vi "BenchC2_DEV_v15_3.vi"() -> ()   [LabVIEW 2017]
uses:
  x64/Debug/BERTTA.dll
panel:
  out "Started:":string
  in  "SHUTDOWN":bool
  in  "MASTER CONTROL":bool
  in  "Tab Control":T1(tab)
  out "Output File":path caption="selected path"
  in  "Browse folder":path=path "" caption="start path"
  in  "Read Seq":bool
  in  "Save Seq":bool
  in  "Configuration file":path caption="Filename"
  in  "OK Button 2":bool
  out "Boolean":bool
  in  "User (initials)":string
  in  "Project name":string
  in  "Description":string
  out "Led11 12":bool
  out "Led11 11":bool
  out "PUMP1":bool
  out "Target amount":dbl format="Target amount:        %#_g"
  out "Scale weight":dbl format="Scale weight:     %#_4g"
  out "Amount now":dbl format="Amount now:      %#_4g"
  out "Flow rate":dbl format="Flow rate:                   %#_4g"
  out "Time to target":dbl format="Time to target:     %<%H:%M:%S>t"
  out "Current step":dbl format="Current step:              %#_g"
  out "Target":dbl format="Target:                %#_4g"
  out "Amount now":dbl format="Amount now:    %#_4g"
  out "Amount now":dbl
  out "Target":dbl
  out "Current step":dbl
  out "Time to target":dbl format="%<%H:%M:%S>t"
  out "Flow rate":dbl
  out "Amount now":dbl
  out "Scale weight":dbl
  out "Target amount":dbl
  out "PUMP2":bool
  out "Sensor OK 6":bool
  out "Sensor OK 5":bool
  out "Sensor OK 4":bool
  out "Sensor OK 3":bool
  in  "OK Button":bool
  in  "Add comment":string
  out "Tr":dbl format="Tr:              %#_4g"
  out "Tj in":dbl format="Tj in:        %#_4g"
  out "Tj out":dbl format="Tj out:        %#_4g"
  out "T set":dbl format="T set:          %#_g"
  out "Current step":i32 format="Current step:  %.0f"
  out "RPM":dbl format="RPM:          %#_g"
  out "Torque 2":dbl format="Torque:      %#_g"
  out "PUMP3":bool
  out "Target amount":dbl
  out "Scale weight":dbl
  out "Amount now":dbl
  out "Flow rate":dbl
  out "Time to target":dbl format="%<%H:%M:%S>t"
  out "Current step":dbl
  out "Target":dbl
  out "Amount now":dbl
  out "Waveform Chart 5":dynamicdata(graph)
  out "Waveform Chart 6":dynamicdata(graph)
  out "Waveform Chart 7":dynamicdata(graph)
  out "Led11 10":bool
  out "T external 3":dbl format="T (S2):       %#_4g"
  out "Table":string[][](table)=[["14.8.2017 18.06.59", "0,000000", "417,670000", "-0,150000", "1,000000", "22,220000", "23,366837", "23,574959", "23,985852", "23,690000", "240,000000", "4,000000", "0,000000", "397,000000", "-397,000000", "1,000000"], ["14.8.2017 18.07.06", "0,000000", "417,640000", "-0,120000", "1,000000", "22,220000", "23,763115", "23,906257", "23,985694", "23,680000", "240,000000", "4,000000", "0,000000", "397,000000", "-397,000000", "1,000000"], ["14.8.2017 18.07.13", "0,000000", "417,640000", "-0,120000", "1,000000", "22,220000", "23,965922", "24,013440", "23,984906", "23,670000", "240,000000", "4,100000", "3,000000", "397,000000", "-397,000000", "1,000000"], ["14.8.2017 18.07.21", "0,000000", "417,640000", "-0,120000", "1,000000", "22,220000", "23,943860", "23,900110", "23,987113", "23,670000", "240,000000", "4,000000", "0,000000", "397,000000", "-397,000000", "1,000000"], ["14.8.2017 18.07.28", "0,000000", "417,640000", "-0,120000", "1,000000", "22,220000", "23,736328", "23,600018", "23,989004", "23,660000", "240,000000", "4,000000", "0,000000", "397,000000", "-397,000000", "1,000000"], ["14.8.2017 18.07.36", "0,000000", "417,640000", "-0,120000", "1,000000", "22,220000", "23,480910", "23,324538", "23,991053", "23,660000", "240,000000", "4,000000", "0,000000", "397,000000", "-397,000000", "1,000000"], ["14.8.2017 18.07.43", "0,000000", "417,640000", "-0,120000", "2,000000", "22,220000", "23,195579", "23,008270", "23,999093", "23,650000", "240,000000", "4,000000", "0,000000", "397,000000", "-397,000000", "1,000000"], ["14.8.2017 18.07.51", "0,000000", "417,650000", "-417,650000", "1,000000", "22,220000", "22,862541", "22,649021", "24,003979", "23,650000", "240,000000", "4,000000", "0,000000", "397,000000", "-397,000000", "2,000000"], ["14.8.2017 18.07.58", "0,000000", "417,640000", "0,010000", "1,000000", "22,220000", "22,541353", "22,354878", "24,005398", "23,650000", "240,000000", "4,000000", "0,000000", "397,000000", "-397,000000", "1,000000"], ["14.8.2017 18.08.06", "0,000000", "417,640000", "0,010000", "1,000000", "22,220000", "22,347931", "22,253738", "24,007605", "23,640000", "240,000000", "4,100000", "0,000000", "397,000000", "-397,000000", "1,000000"], ["14.8.2017 18.08.13", "0,000000", "417,640000", "0,010000", "1,000000", "22,220000", "22,329030", "22,302102", "24,006028", "23,640000", "240,000000", "4,000000", "0,000000", "395,820000", "-395,820000", "1,000000"], ["14.8.2017 18.08.20", "0,000000", "417,640000", "0,010000", "1,000000", "22,220000", "22,466849", "22,511320", "24,002403", "23,630000", "240,000000", "4,000000", "0,000000", "395,830000", "-0,010000", "1,000000"], ["14.8.2017 18.08.28", "0,000000", "417,640000", "0,010000", "1,000000", "22,220000", "22,707062", "22,835101", "24,000984", "23,620000", "240,000000", "4,000000", "0,000000", "395,830000", "-0,010000", "1,000000"], ["14.8.2017 18.08.35", "0,000000", "417,640000", "0,010000", "1,000000", "22,220000", "23,054104", "23,232979", "24,001299", "23,600000", "240,000000", "4,000000", "0,000000", "395,830000", "-0,010000", "1,000000"], ["14.8.2017 18.08.43", "0,000000", "417,640000", "0,010000", "1,000000", "22,220000", "23,412371", "23,522793", "24,002560", "23,590000", "240,000000", "4,000000", "0,000000", "395,820000", "0,000000", "1,000000"], ["14.8.2017 18.08.51", "0,000000", "417,640000", "0,010000", "1,000000", "22,220000", "23,596247", "23,656125", "24,003821", "23,580000", "240,000000", "4,000000", "0,000000", "395,820000", "0,000000", "1,000000"]]
  out "LED_5":bool
  out "LED_4":bool
  in  "PAUSE/RUN 4":bool
  in  "TEMP RAMP":dbl[][](array[numeric])
  out "LED_3":bool
  out "LED_2":bool
  out "LED_1":bool
  out "LED_MANUAL":bool
  in  "Reset 6":bool
  in  "Manual/Ramp":bool=TRUE
  in  "Sensor selector":bool=TRUE
  in  "Tr/Tj mode selector":bool=TRUE
  out "LED STOP":bool
  in  "Failsafe":dbl=20.0 format="Failsafe temperature:            %#_g"
  out "Current temp":dbl format="Current temperature S1:       %#_4g"
  out "Sensor OK":bool
  out "T external 2":dbl format="Current temperature S2:       %#_4g"
  in  "OK Button 3":bool
  out "Waveform Chart":dynamicdata(graph)
  in  "X scale":i64(slide)=50 scale=0.0..100.0
  out "Led11 7":bool
  out "Led11 6":bool
  out "Led11 7":bool
  out "Led11 6":bool
  out "Led5 7":bool
  out "Led4 6":bool
  out "Waveform Chart 18":dynamicdata(graph)
  in  "PAUSE/RUN 3":bool
  in  "Tube select 3":u32(ring) items=["Big tube", "Double big tube", "Medium tube", "Small tube"]
  in  "Reset 8":bool
  out "Led11 9":bool
  in  "?":bool
  in  "Grams / min 3":dbl
  out "RPM 3":dbl format="%_4f"
  out "Flow rate (g/min) 3":dbl
  out "Scale reading 3":dbl
  out "Step amount now 3":dbl
  out "Total amount now 3":dbl
  out "Elapsed / step 3":dbl format="%<%H:%M:%S>t"
  out "Time to target 3":dbl format="%<%H:%M:%S>t"
  out "Led5 5":bool
  out "Led4 5":bool
  out "Led3 5":bool
  out "Led2 5":bool
  out "Led1 5":bool
  in  "PumpSeq 6":dbl[][](array[numeric])=[[0.0, 0.0, 0.0, 0.0, 0.0, 0.0, 0.0, 0.0, 0.0, 0.0], [0.0, 0.0, 0.0, 0.0, 0.0, 0.0, 0.0, 0.0, 0.0, 0.0], [0.0, 0.0, 0.0, 0.0, 0.0, 0.0, 0.0, 0.0, 0.0, 0.0], [0.0, 0.0, 0.0, 0.0, 0.0, 0.0, 0.0, 0.0, 0.0, 0.0], [0.0, 0.0, 0.0, 0.0, 0.0, 0.0, 0.0, 0.0, 0.0, 0.0], [0.0, 0.0, 0.0, 0.0, 0.0, 0.0, 0.0, 0.0, 0.0, 0.0], [0.0, 0.0, 0.0, 0.0, 0.0, 0.0, 0.0, 0.0, 0.0, 0.0], [0.0, 0.0, 0.0, 0.0, 0.0, 0.0, 0.0, 0.0, 0.0, 0.0], [0.0, 0.0, 0.0, 0.0, 0.0, 0.0, 0.0, 0.0, 0.0, 0.0], [0.0, 0.0, 0.0, 0.0, 0.0, 0.0, 0.0, 0.0, 0.0, 0.0]]
  out "Led11 8":bool
  in  "PAUSE/RUN 2":bool
  in  "Tube select 2":u32(ring) items=["Big tube", "Double big tube", "Medium tube", "Small tube"]
  out "Led11 7":bool
  in  "?":bool
  in  "Grams / min 2":dbl
  out "RPM 2":dbl format="%_4f"
  out "Flow rate (g/min) 2":dbl
  out "Scale reading 2":dbl
  out "Step amount now 2":dbl
  out "Total amount now 2":dbl
  out "Elapsed / step 2":dbl format="%<%H:%M:%S>t"
  out "Time to target 2":dbl format="%<%H:%M:%S>t"
  out "Led5 4":bool
  out "Led4 4":bool
  out "Led3 4":bool
  out "Led2 4":bool
  out "Led1 4":bool
  in  "PumpSeq 5":dbl[][](array[numeric])=[[0.0, 0.0, 0.0, 0.0, 0.0, 0.0, 0.0, 0.0, 0.0, 0.0], [0.0, 0.0, 0.0, 0.0, 0.0, 0.0, 0.0, 0.0, 0.0, 0.0], [0.0, 0.0, 0.0, 0.0, 0.0, 0.0, 0.0, 0.0, 0.0, 0.0], [0.0, 0.0, 0.0, 0.0, 0.0, 0.0, 0.0, 0.0, 0.0, 0.0], [0.0, 0.0, 0.0, 0.0, 0.0, 0.0, 0.0, 0.0, 0.0, 0.0], [0.0, 0.0, 0.0, 0.0, 0.0, 0.0, 0.0, 0.0, 0.0, 0.0], [0.0, 0.0, 0.0, 0.0, 0.0, 0.0, 0.0, 0.0, 0.0, 0.0], [0.0, 0.0, 0.0, 0.0, 0.0, 0.0, 0.0, 0.0, 0.0, 0.0], [0.0, 0.0, 0.0, 0.0, 0.0, 0.0, 0.0, 0.0, 0.0, 0.0], [0.0, 0.0, 0.0, 0.0, 0.0, 0.0, 0.0, 0.0, 0.0, 0.0]]
  out "Led11 6":bool
  in  "Reset 7":bool
  in  "PAUSE/RUN":bool
  in  "Tube select":u32(ring) items=["Big tube", "Double big tube", "Medium tube", "Small tube"]
  out "Led11 5":bool
  out "RPM":dbl format="RPM                      %_4f"
  out "Flow rate (g/min)":dbl format="Flow rate               %#_g"
  out "Scale reading":dbl format="Scale reading       %#_g"
  out "Step amount now":dbl format="Step amount       %#_g"
  out "Total amount now":dbl format="Total amount      %#_g"
  out "Elapsed / step":dbl format="Elapsed / step      %<%H:%M:%S>t"
  out "Time to target":dbl format="Time to target     %<%H:%M:%S>t"
  out "Led5 3":bool
  out "Led4 3":bool
  out "Led3 3":bool
  out "Led2 3":bool
  out "Led1 3":bool
  in  "PumpSeq 4":dbl[][](array[numeric])=[[0.0, 0.0, 0.0, 0.0, 0.0, 0.0, 0.0, 0.0, 0.0, 0.0], [0.0, 0.0, 0.0, 0.0, 0.0, 0.0, 0.0, 0.0, 0.0, 0.0], [0.0, 0.0, 0.0, 0.0, 0.0, 0.0, 0.0, 0.0, 0.0, 0.0], [0.0, 0.0, 0.0, 0.0, 0.0, 0.0, 0.0, 0.0, 0.0, 0.0], [0.0, 0.0, 0.0, 0.0, 0.0, 0.0, 0.0, 0.0, 0.0, 0.0], [0.0, 0.0, 0.0, 0.0, 0.0, 0.0, 0.0, 0.0, 0.0, 0.0], [0.0, 0.0, 0.0, 0.0, 0.0, 0.0, 0.0, 0.0, 0.0, 0.0], [0.0, 0.0, 0.0, 0.0, 0.0, 0.0, 0.0, 0.0, 0.0, 0.0], [0.0, 0.0, 0.0, 0.0, 0.0, 0.0, 0.0, 0.0, 0.0, 0.0], [0.0, 0.0, 0.0, 0.0, 0.0, 0.0, 0.0, 0.0, 0.0, 0.0]]
  in  "?":bool
  in  "Grams / min":dbl format="Manual g/min:  %#_g"
  out "Led11 4":bool
  in  "Reset 5":bool
  in  "OK Button 4":bool
  out "Waveform Chart 16":dynamicdata(graph)
  in  "OK Button 5":bool
  out "Waveform Chart 17":dynamicdata(graph)
  in  "OK Button 6":bool
  in  "PAUSE/RUN 5":bool
  in  "?":bool
  in  "Scale port":dbl=5.0
  out "Waveform Chart 15":dynamicdata(graph)
  in  "OK Button 8":bool
  in  "PAUSE/RUN 6":bool
  in  "Set RPM":i32
  in  "Remote / Manual":bool
  out "RPM":dbl
  out "Torque":dbl
  out "Waveform Chart 4":dynamicdata(graph)
  in  "OK Button 7":bool
  in  "CDAQ Temp Control":tag="cDAQ9188XT-1C3BF12Mod1"
  in  "CDAQ PAM Control":tag="cDAQ9188XT-1C3BF12Mod1"
  in  "PORT PUMP2":i32 format="PUMP 2 PORT:  %.0f"
  in  "PORT PUMP3":i32 format="PUMP 3 PORT:  %.0f"
  in  "PORT PUMP1":i32 format="PUMP 1 PORT:  %.0f"
  in  "Save PortDev":bool
  in  "LAUDA":i32 format="LAUDA PORT:  %.0f"
  in  "HEIDOLPH":i32 format="HEIDOLPH PORT:  %.0f"
  in  "SCALE1":i32 format="SCALE 1 PORT:  %.0f"
  in  "SCALE2":i32 format="SCALE 2 PORT:  %.0f"
  in  "SCALE 3":i32 format="SCALE 3 PORT:  %.0f"
  # "PUMP & SCALE 1"
  # "PUMP & SCALE 2"
  # "PUMP & SCALE 3"
  # "STEP"
  # "STEP"
  # "STEP"
  # "TOTAL"
  # "TOTAL"
  # "TOTAL"
  # "Temperature sensor:"
  # "Manual control:"
  # "MANUAL"
  # "RAMP"
  # "Temp Target       Time Target          Wait Time"
  # "STOP"
  # "g              min"
  # "g              min"
  # "g              min"
  # "PAM control"
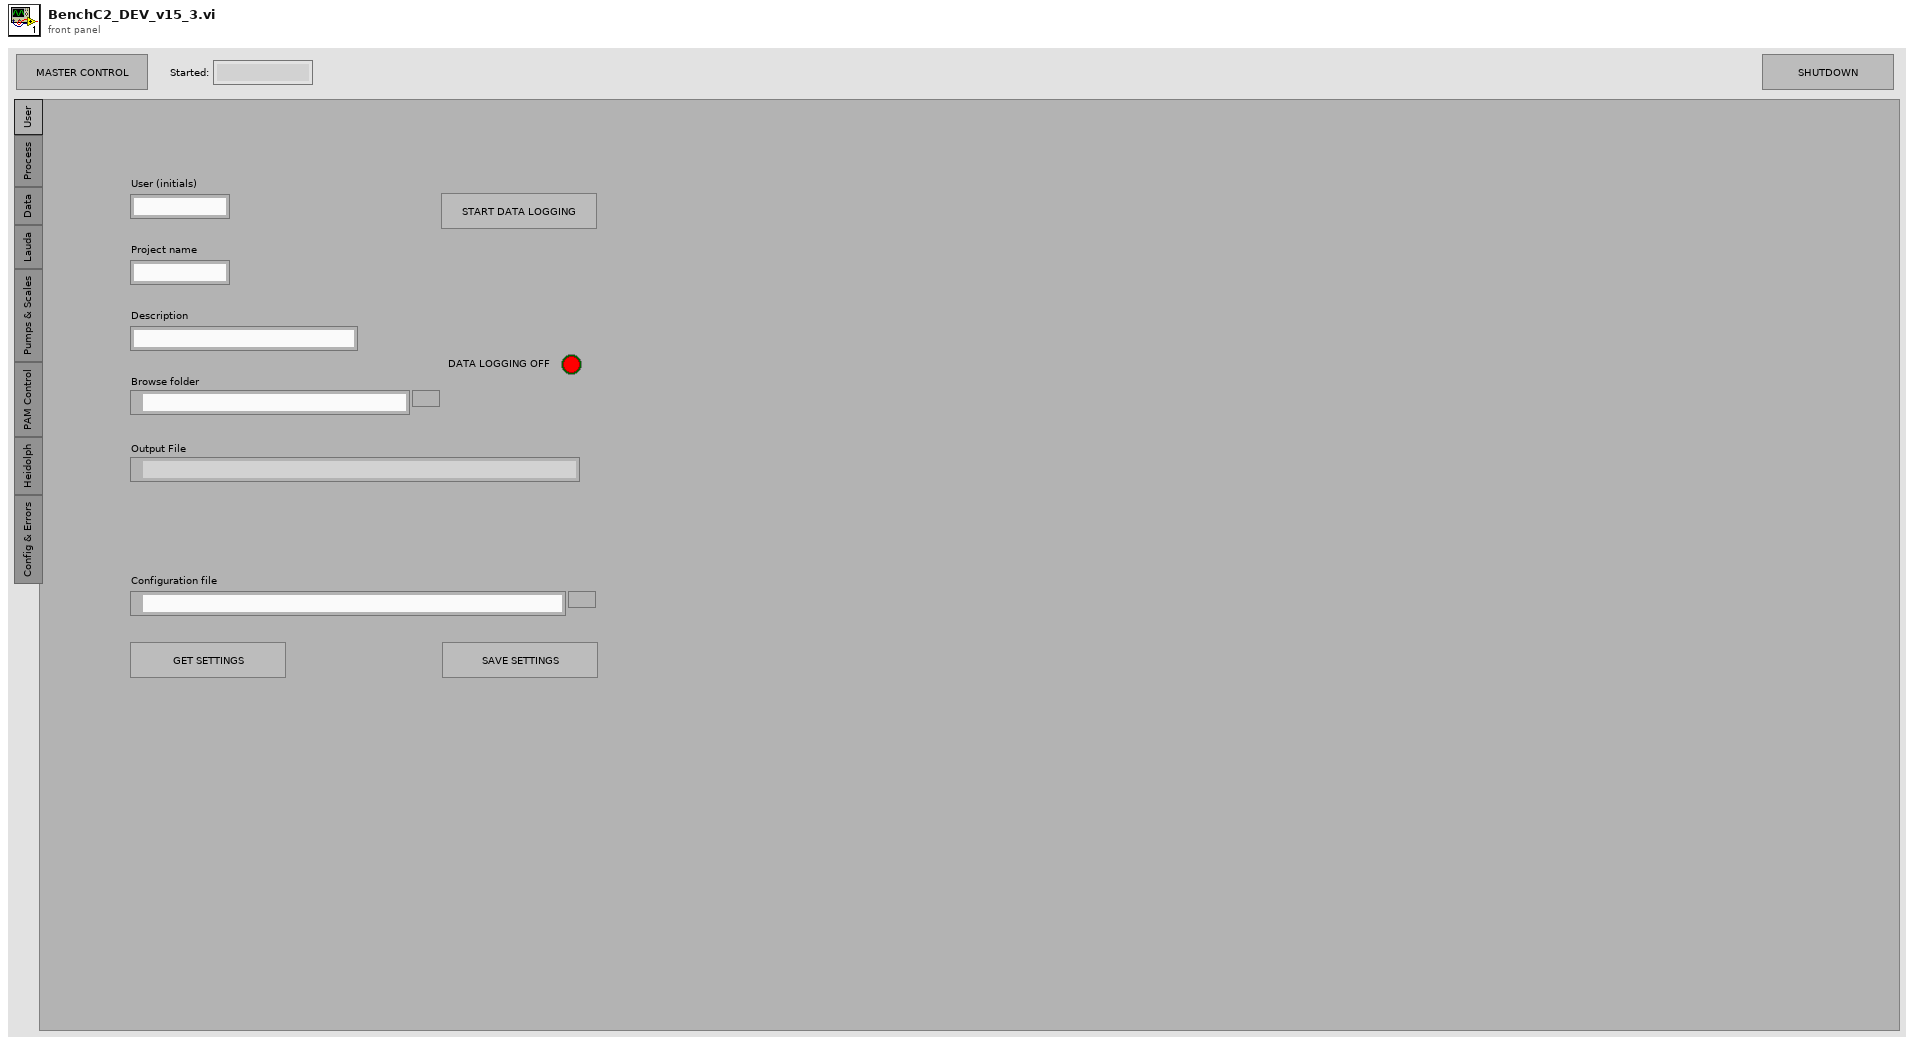
[diagram p1: front panel]
types:
  T1 = enum32{"User", "Process", "Data", "Lauda", "Pumps & Scales", "PAM Control", "Heidolph", "Config & Errors"}
diagram:
  n1 = while {
    i -> [w227]
    stop <- FALSE stop-if-true
    w31 = i64 1000 ("y")
    # "TARKISTA: negatiiviset lämpötilat, toimivatko"
    # "X-skaalaus puuttuu"
    # "SCALE & PUMP 1"
    # "SCALE & PUMP 3"
    n2 = And(x="PAUSE/RUN 6", y="MASTER CONTROL") -> (x .and. y?=w8:bool)
    n3 = feedback #1() -> (w36:dbl[][])  [unwired: 1 in]
    n4 = Select(t="TEMP RAMP", s="Reset 6", f=w36) -> (s? t:f=w37:dbl[][])
    n5 = feedback-in #1(w37) -> ()
    n6 = Initialize Array(0.0 ("element"), 5 ("dimension size"), 3 ("dimension size")) -> (w81:dbl[][])
    n7 = Select(t="Set RPM", s=w8, f=10) -> (s? t:f=w12:i32)
    n8 = Not(x="MASTER CONTROL") -> (.not. x?=w280:bool)
    n9 = Replace Array Subset(array=w81, new element=w36, index (row)=0, index (col)=0 ("disabled index (col)")) -> (w55:dbl[][])
    n10 = control-ref of="This VI"() -> (w4:refnum<vi>)
    n11 = Multiply(x="X scale", y=w31) -> (x*y=w32:i64)
    n12 = Boolean To (0,1)(Boolean=w280) -> (0, 1=w281:i16)
    n13 = Add(x=w32, y=w31) -> (x+y=w27:i64)
    n14 = for {
      N: w281 -> [_]
      n15 = Get Date/Time String(want seconds? (F)=TRUE) -> (time string=→"Started:":string)  [unwired: 2 in, 1 out]
    }
    n16 = feedback #2() -> (w30:i64)  [unwired: 1 in]
    n17 = feedback-in #2(w27) -> ()
    n18 = Boolean To (0,1)(Boolean="Sensor selector") -> (0, 1=w63:i16)
    n19 = Boolean To (0,1)(Boolean="SHUTDOWN") -> (0, 1=w2:i16)
    n20 = call "shutdown sequence.vi"("SHUTDOWN"="SHUTDOWN", "VI in"=w4) -> ()  [unwired: 10 in]
    n21 = Not Equal?(x=w30, y=w27) -> (x != y?=w29:bool)
    n22 = property on="Waveform Chart" class="WFChart (strict)"() -> ("History Data"=w34:dynamicdata[])  [unwired: 2 in, 2 out]
    n23 = Boolean To (0,1)(Boolean=w29) -> (0, 1=w26:i16)
    n24 = Array Size(array=w34) -> (size(s)=w28:i32)
    n25 = Boolean To (0,1)(Boolean="SHUTDOWN") -> (0, 1=w5:i16)
    n26 = Boolean To (0,1)(Boolean="Tr/Tj mode selector") -> (0, 1=w75:i16)
    n27 = formula code="int SensorLED1 = 0, SensorLED0 = 0, ModeLED1 = 0, ModeLED0 = 0;\nif(Sensor==1) SensorLED1 = 1;\nif(Sensor==0) SensorLED0 = 1;\nif(Tr_Tj==1) ModeLED1 = 1;\nif(Tr_Tj==0) ModeLED0 = 1;"("Tr_Tj"=w75, "Sensor"=w63) -> ("SensorLED1"=w73:i32, "SensorLED0"=w71:i32, "ModeLED1"=w56:i32, "ModeLED0"=w66:i32)
    n28 = Equal?(x=w73, y=1.0) -> (x = y?=→"Sensor OK 3":bool)
    n29 = Equal?(x=w71, y=1.0) -> (x = y?=→"Sensor OK 4":bool)
    n30 = for {
      N: w26 -> [_]
      tunnel: w28 -> [w288]
      tunnel: w27 -> [w287]
      n31 = Add(x=w288, y=w287) -> (x+y=w286:i64)
      n32 = property on="Waveform Chart" class="WFChart (strict)"("XScale.Maximum"=w286) -> ()  [unwired: 2 in, 2 out]
    }
    n33 = call "MReadRS232_2.vi"("port1"="LAUDA", "dev1"=1, "port2"="LAUDA", "dev2"=2, "port3"="HEIDOLPH", "dev7"=5, "dev8"=0, "port7"="SCALE 3", "port8"=0, "dev5"=5, "port5"="SCALE1", "dev4"=4, "dev6"=5, "port6"="SCALE2", "port4"="HEIDOLPH", "dev3"=3) -> ("params"=w99:dbl[])  [unwired: 10 in, 1 out]
    n34 = call "HEI_CTRL.vi"("shutdown"=w5, "Set RPM"=w12, "Remote / Manual"="Remote / Manual", "port3"="HEIDOLPH") -> ()  [unwired: 8 in]
    n35 = And(x="MASTER CONTROL", y="PAUSE/RUN 4") -> (x .and. y?=w101:bool)
    n36 = Index Array(array=w55, index (col)=2 ("disabled index (col)")) -> (element=w88:dbl[])  [unwired: 1 in]
    n37 = Equal?(x=w56, y=1.0) -> (x = y?=→"Sensor OK 6":bool)
    n38 = Equal?(x=w66, y=1.0) -> (x = y?=→"Sensor OK 5":bool)
    n39 = Boolean To (0,1)(Boolean=w101) -> (0, 1=w100:i16)
    n40 = Boolean To (0,1)(Boolean="Manual/Ramp") -> (0, 1=w102:i16)
    n41 = Boolean To (0,1)(Boolean="Reset 6") -> (0, 1=w104:i16)
    n42 = Build Array("LAUDA", "HEIDOLPH", "SCALE1", "SCALE2", "SCALE 3", "PORT PUMP1", "PORT PUMP2", "PORT PUMP3") -> (w42:i32[])
    n43 = Index Array(array=w55, index (col)=1 ("disabled index (col)")) -> (element=w90:dbl[])  [unwired: 1 in]
    n44 = Index Array(array=w55, index (col)=0 ("disabled index (col)")) -> (element=w91:dbl[])  [unwired: 1 in]
    n45 = call "LaudaDAQ.vi"("device name"="CDAQ Temp Control") -> (1:"Tj out"=→"Tj out":dbl, "data"=w264:dynamicdata, "Sensor OK"=→"Sensor OK":bool, 4:"Tj out"=→"Tj in":dbl, "T external 2"=w7:dbl)  [unwired: 5 in, 1 out]
    "T external 2" <- w7
    "T external 3" <- w7
    n46 = call "Ramp_Lauda_v3.vi"("manual"=w102, "Tr_Tj"=w75, "shutdown"=w2, "S1_S2"=w63, "Tr"=w99, "T_fail"="Failsafe", "enable"=w100, "time_set"=w90, "reset"=w104, "time_wait"=w88, "T_S2"=w7, "port"="LAUDA", "T_sp"=w91) -> ("LED_1"=→"LED_1":bool, "LED_manual"=→"LED_MANUAL":bool, "LED_2"=→"LED_2":bool, "step"=w53:dbl, "LED_stop"=→"LED STOP":bool, "LED_3"=→"LED_3":bool, "LED 4"=→"LED_4":bool, "LED 5"=→"LED_5":bool, "setpoint"=w50:dbl, "Tr_out"=w98:dbl, "T int"=w97:dbl)  [unwired: 2 in, 2 out]
    "Tr" <- w98
    "T set" <- w50
    "Current temp" <- w98
    n47 = Boolean To (0,1)(Boolean="Save PortDev") -> (0, 1=w230:i16)
    n48 = for {
      N: w230 -> [_]
      tunnel: w42 -> [w334]
      tunnel: "Save PortDev" -> [w335]
      n49 = call "Convert to Dynamic Data"("Array"=w334) -> ("Dynamic Data Type"=w333:dynamicdata)  [unwired: 3 in]
      n50 = call "Write To Measurement File3"("Signals"=w333, "Reset"=w335) -> ()  [unwired: 15 in, 3 out]
    }
    n51 = Add(x=w53, y=1.0) -> (x+y=→"Current step":dbl)
    n52 = Less?(x=w227, y=1.0) -> (x < y?=w225:bool)
    n53 = Index Array(array=w99, index=3) -> (element=w218:dbl)
    "RPM" <- w218
    "RPM" <- w218
    n54 = Index Array(array=w99, index=2) -> (element=w220:dbl)
    n55 = Boolean To (0,1)(Boolean=w225) -> (0, 1=w226:i16)
    n56 = Divide(x=w220, y=10.0) -> (x/y=w217:dbl)
    "Torque" <- w217
    "Torque 2" <- w217
    n57 = for {
      N: w226 -> [_]
      tunnel: w225 -> [w328]
      n58 = while {
        tunnel: [w331] -> w327
        tunnel: w328 -> [w329]
        stop <- w332 stop-if-true
        n59 = call "Read From Measurement File2"("Enable"=TRUE, "Reset"=w329) -> ("Signals"=w331:dynamicdata, "EOF?"=w332:bool)  [unwired: 4 in, 4 out]
      }
      n60 = call "Convert from Dynamic Data2"("Dynamic Data Type"=w327) -> ("Array"=w313:dbl[])  [unwired: 3 in]
      n61 = Index Array(array=w313, index=0) -> (element=w320:dbl)
      n62 = Index Array(array=w313, index=1) -> (element=w319:dbl)
      n63 = Index Array(array=w313, index=2) -> (element=w318:dbl)
      n64 = Index Array(array=w313, index=3) -> (element=w317:dbl)
      n65 = Index Array(array=w313, index=4) -> (element=w316:dbl)
      n66 = Index Array(array=w313, index=5) -> (element=w310:dbl)
      n67 = Index Array(array=w313, index=6) -> (element=w312:dbl)
      n68 = Index Array(array=w313, index=7) -> (element=w311:dbl)
      n69 = property on="LAUDA" class="DigNum (strict)"("Val(Sgnl)"=w320) -> ()  [unwired: 2 in, 2 out]
      n70 = property on="HEIDOLPH" class="DigNum (strict)"("Val(Sgnl)"=w319) -> ()  [unwired: 2 in, 2 out]
      n71 = property on="SCALE1" class="DigNum (strict)"("Val(Sgnl)"=w318) -> ()  [unwired: 2 in, 2 out]
      n72 = property on="SCALE2" class="DigNum (strict)"("Val(Sgnl)"=w317) -> ()  [unwired: 2 in, 2 out]
      n73 = property on="SCALE 3" class="DigNum (strict)"("Val(Sgnl)"=w316) -> ()  [unwired: 2 in, 2 out]
      n74 = property on="PORT PUMP2" class="DigNum (strict)"("Val(Sgnl)"=w312) -> ()  [unwired: 2 in, 2 out]
      n75 = property on="PORT PUMP3" class="DigNum (strict)"("Val(Sgnl)"=w311) -> ()  [unwired: 2 in, 2 out]
      n76 = property on="PORT PUMP1" class="DigNum (strict)"("Val(Sgnl)"=w310) -> ()  [unwired: 2 in, 2 out]
    }
    n77 = Merge Signals(w218, w217) -> (w216:dynamicdata)
    "Waveform Chart 4" <- w216
    "Waveform Chart 6" <- w216
    n78 = Boolean To (0,1)(Boolean="OK Button 3") -> (0, 1=w245:i16)
    n79 = for {
      N: w245 -> [_]
      n80 = property on="Waveform Chart" class="WFChart (strict)"("History Data"=dynamicdata[] []) -> ()  [unwired: 2 in, 2 out]
    }
    n81 = Merge Signals(w50, w98, w97, w264) -> (w265:dynamicdata)
    "Waveform Chart" <- w265
    "Waveform Chart 5" <- w265
    n82 = Boolean To (0,1)(Boolean="OK Button 4") -> (0, 1=w243:i16)
    n83 = for {
      N: w243 -> [_]
      n84 = property on="Waveform Chart 18" class="WFChart (strict)"("History Data"=dynamicdata[] []) -> ()  [unwired: 2 in, 2 out]
    }
    n85 = Boolean To (0,1)(Boolean="?") -> (0, 1=w209:i16)
    n86 = Boolean To (0,1)(Boolean="PAUSE/RUN") -> (0, 1=w182:i16)
    n87 = Boolean To (0,1)(Boolean="MASTER CONTROL") -> (0, 1=w207:i16)
    n88 = Boolean To (0,1)(Boolean="Reset 5") -> (0, 1=w202:i16)
    n89 = Boolean To (0,1)(Boolean="OK Button 5") -> (0, 1=w61:i16)
    n90 = And(x=w207, y=w182) -> (x .and. y?=w206:i16)
    n91 = for {
      N: w61 -> [_]
      n92 = property on="Waveform Chart 16" class="WFChart (strict)"("History Data"=dynamicdata[] []) -> ()  [unwired: 2 in, 2 out]
    }
    n93 = Index Array(array="PumpSeq 4", index (col)=0) -> (element=w204:dbl[])  [unwired: 1 in]
    n94 = Index Array(array="PumpSeq 4", index (col)=1) -> (element=w205:dbl[])  [unwired: 1 in]
    n95 = call "PID_Flow Ctrl_2 P1.vi"("weight"=w99, "Setpoint_W"=w204, "Setpoint_T"=w205, "FrManual"="Grams / min", "enable"=w206, "manual"=w209, "reset"=w202, "tube"="Tube select") -> ("elapsed_step"=→"Elapsed / step":dbl, "total_target"=→"Target":dbl, "Setpoint_W"=→"Target amount":dbl, "LED_stop"=w181:bool, "RPM"=w203:dbl, "LED1"=→"Led1 3":bool, "LED4"=→"Led4 3":bool, "LED2"=→"Led2 3":bool, "step_amount"=→"Amount now" →"Step amount now":dbl, "LED3"=→"Led3 3":bool, "LED5"=→"Led5 3":bool, "weight"=w192:dbl, "time_to_target"=→"Time to target" →"Time to target":dbl, "LED6"=→"Led4 6":bool, "LED7"=→"Led5 7":bool, "PumpCTRL"=w186:dbl, "step"=→"Current step":dbl, "LED_manual"=→"Led11 5" →"Led11 10":bool, "FR"=w183:dbl)  [unwired: 1 in]
    "Flow rate" <- w183
    "Scale weight" <- w192
    "Led11 4" <- w181
    "Scale reading" <- w192
    "Flow rate (g/min)" <- w183
    "RPM" <- w203
    n96 = Merge Signals(w192, w183) -> (w62:dynamicdata)
    "Waveform Chart 18" <- w62
    n97 = Greater?(x=w186, y=70.0) -> (0:→"PUMP1":bool)
    n98 = Multiply(x=-1.0, y=w192) -> (x*y=→"Amount now" →"Total amount now":dbl)
    n99 = Boolean To (0,1)(Boolean="OK Button 6") -> (0, 1=w59:i16)
    n100 = for {
      N: w59 -> [_]
      n101 = property on="Waveform Chart 17" class="WFChart (strict)"("History Data"=dynamicdata[] []) -> ()  [unwired: 2 in, 2 out]
    }
    n102 = And(x="PAUSE/RUN", y=w181) -> (x .and. y?=w179:bool)
    n103 = feedback #3() -> (w180:bool)  [unwired: 1 in]
    n104 = feedback-in #3(w179) -> ()
    n105 = Not Equal?(x=w180, y=w179) -> (x != y?=w178:bool)
    n106 = Boolean To (0,1)(Boolean=w178) -> (0, 1=w177:i16)
    n107 = for {
      N: w177 -> [_]
      n108 = property on="PAUSE/RUN" class="Bool (strict)"("Val(Sgnl)"=FALSE ("Value (Signaling)")) -> ()  [unwired: 2 in, 2 out]
    }
    n109 = Boolean To (0,1)(Boolean="OK Button 7") -> (0, 1=w241:i16)
    n110 = for {
      N: w241 -> [_]
      n111 = property on="Waveform Chart 4" class="WFChart (strict)"("History Data"=dynamicdata[] []) -> ()  [unwired: 2 in, 2 out]
    }
    n112 = Boolean To (0,1)(Boolean="OK Button 8") -> (0, 1=w213:i16)
    n113 = for {
      N: w213 -> [_]
      n114 = property on="Waveform Chart 15" class="WFChart (strict)"("History Data"=dynamicdata[] []) -> ()  [unwired: 2 in, 2 out]
    }
    n115 = Index Array(array="PumpSeq 5", index (col)=0) -> (element=w160:dbl[])  [unwired: 1 in]
    n116 = Index Array(array="PumpSeq 5", index (col)=1) -> (element=w161:dbl[])  [unwired: 1 in]
    n117 = Boolean To (0,1)(Boolean="PAUSE/RUN 2") -> (0, 1=w175:i16)
    n118 = Boolean To (0,1)(Boolean="MASTER CONTROL") -> (0, 1=w176:i16)
    n119 = And(x=w176, y=w175) -> (x .and. y?=w174:i16)
    n120 = Boolean To (0,1)(Boolean="Reset 7") -> (0, 1=w165:i16)
    n121 = Boolean To (0,1)(Boolean="?") -> (0, 1=w167:i16)
    n122 = call "PID_Flow Ctrl_2 P2.vi"("weight"=w99, "Setpoint_W"=w160, "Setpoint_T"=w161, "FrManual"="Grams / min 2", "enable"=w174, "manual"=w167, "reset"=w165, "tube"="Tube select 2") -> ("elapsed_step"=→"Elapsed / step 2":dbl, "total_target"=→"Target":dbl, "Setpoint_W"=→"Target amount":dbl, "LED_stop"=w143:bool, "RPM"=w148:dbl, "LED1"=→"Led1 4":bool, "LED4"=→"Led4 4":bool, "LED2"=→"Led2 4":bool, "step_amount"=→"Amount now" →"Step amount now 2":dbl, "LED3"=→"Led3 4":bool, "LED5"=→"Led5 4":bool, "weight"=w112:dbl, "time_to_target"=→"Time to target" →"Time to target 2":dbl, "LED6"=→"Led11 6":bool, "LED7"=→"Led11 7":bool, "PumpCTRL"=w151:dbl, "step"=→"Current step":dbl, "LED_manual"=→"Led11 7" →"Led11 11":bool, "FR"=w149:dbl)  [unwired: 1 in]
    "Scale weight" <- w112
    "Flow rate" <- w149
    "Led11 6" <- w143
    "Scale reading 2" <- w112
    "Flow rate (g/min) 2" <- w149
    "RPM 2" <- w148
    n123 = Merge Signals(w112, w149) -> (w150:dynamicdata)
    "Waveform Chart 16" <- w150
    n124 = Multiply(x=w112, y=-1.0) -> (x*y=→"Amount now" →"Total amount now 2":dbl)
    n125 = And(x="PAUSE/RUN 2", y=w143) -> (x .and. y?=w146:bool)
    n126 = Greater?(x=w151, y=70.0) -> (0:→"PUMP2":bool)
    n127 = feedback #4() -> (w147:bool)  [unwired: 1 in]
    n128 = feedback-in #4(w146) -> ()
    n129 = Not Equal?(x=w147, y=w146) -> (x != y?=w145:bool)
    n130 = Boolean To (0,1)(Boolean=w145) -> (0, 1=w144:i16)
    n131 = for {
      N: w144 -> [_]
      n132 = property on="PAUSE/RUN 2" class="Bool (strict)"("Val(Sgnl)"=FALSE ("Value (Signaling)")) -> ()  [unwired: 2 in, 2 out]
    }
    n133 = Index Array(array="PumpSeq 6", index (col)=0) -> (element=w129:dbl[])  [unwired: 1 in]
    n134 = Index Array(array="PumpSeq 6", index (col)=1) -> (element=w130:dbl[])  [unwired: 1 in]
    n135 = Boolean To (0,1)(Boolean="MASTER CONTROL") -> (0, 1=w137:i16)
    n136 = Boolean To (0,1)(Boolean="PAUSE/RUN 3") -> (0, 1=w136:i16)
    n137 = And(x=w137, y=w136) -> (x .and. y?=w135:i16)
    n138 = Boolean To (0,1)(Boolean="?") -> (0, 1=w128:i16)
    n139 = Boolean To (0,1)(Boolean="Reset 8") -> (0, 1=w126:i16)
    n140 = call "PID_Flow Ctrl_2 P3.vi"("weight"=w99, "Setpoint_W"=w129, "Setpoint_T"=w130, "FrManual"="Grams / min 3", "enable"=w135, "manual"=w128, "reset"=w126, "tube"="Tube select 3") -> ("elapsed_step"=→"Elapsed / step 3":dbl, "total_target"=→"Target":dbl, "Setpoint_W"=→"Target amount":dbl, "LED_stop"=w105:bool, "RPM"=w110:dbl, "LED1"=→"Led1 5":bool, "LED4"=→"Led4 5":bool, "LED2"=→"Led2 5":bool, "step_amount"=→"Amount now" →"Step amount now 3":dbl, "LED3"=→"Led3 5":bool, "LED5"=→"Led5 5":bool, "weight"=w111:dbl, "time_to_target"=→"Time to target" →"Time to target 3":dbl, "LED6"=→"Led11 6":bool, "LED7"=→"Led11 7":bool, "PumpCTRL"=w123:dbl, "step"=→"Current step":dbl, "LED_manual"=→"Led11 9" →"Led11 12":bool, "FR"=w116:dbl)  [unwired: 1 in]
    "Scale weight" <- w111
    "Flow rate" <- w116
    "Led11 8" <- w105
    "Scale reading 3" <- w111
    "Flow rate (g/min) 3" <- w116
    "RPM 3" <- w110
    n141 = call "MWriteRS232_1.vi"("PORT PUMP3"="PORT PUMP3", "PORT PUMP2"="PORT PUMP2", "PORT PUMP1"="PORT PUMP1", "PORT LAUDA"="LAUDA", "P3"=w110, "P2"=w148, "P1"=w203, "LAUDA"=w50) -> ()  [unwired: 4 in]
    n142 = call "Convert to Dynamic Data4"("2D Array"="PumpSeq 6") -> ("Dynamic Data Type"=w251:dynamicdata)  [unwired: 3 in]
    n143 = call "Convert to Dynamic Data3"("2D Array"="PumpSeq 5") -> ("Dynamic Data Type"=w252:dynamicdata)  [unwired: 3 in]
    n144 = call "Convert to Dynamic Data2"("2D Array"="PumpSeq 4") -> ("Dynamic Data Type"=w254:dynamicdata)  [unwired: 3 in]
    n145 = Merge Signals(w251, w252, w254) -> (w253:dynamicdata)
    n146 = Greater?(x=w123, y=70.0) -> (0:→"PUMP3":bool)
    n147 = Merge Signals(w111, w116) -> (w115:dynamicdata)
    "Waveform Chart 17" <- w115
    n148 = Boolean To (0,1)(Boolean="Save Seq") -> (0, 1=w250:i16)
    n149 = Multiply(x=w111, y=-1.0) -> (x*y=→"Amount now" →"Total amount now 3":dbl)
    n150 = for {
      N: w250 -> [_]
      tunnel: w253 -> [w376]
      tunnel: "Configuration file" -> [w377]
      tunnel: "Save Seq" -> [w375]
      n151 = call "Write To Measurement File2"("Signals"=w376, "Reset"=w375, "Filename"=w377) -> ()  [unwired: 14 in, 3 out]
    }
    n152 = Merge Signals(w62, w150, w115) -> (w266:dynamicdata)
    n153 = Merge Signals(w192, w112, w111) -> (→"Waveform Chart 7":dynamicdata)
    n154 = And(x="MASTER CONTROL", y=w105) -> (x .and. y?=w108:bool)
    n155 = feedback #5() -> (w109:bool)  [unwired: 1 in]
    n156 = feedback-in #5(w108) -> ()
    n157 = Not Equal?(x=w109, y=w108) -> (x != y?=w107:bool)
    n158 = Boolean To (0,1)(Boolean="Read Seq") -> (0, 1=w249:i16)
    n159 = for {
      N: w249 -> [_]
      tunnel: "Configuration file" -> [w350]
      tunnel: "Read Seq" -> [w349]
      n160 = while {
        tunnel: [w374] -> w370
        tunnel: w350 -> [w373]
        tunnel: w349 -> [w371]
        stop <- w372 stop-if-true
        n161 = call "Read From Measurement File"("Filename"=w373, "Reset"=w371) -> ("Signals"=w374:dynamicdata, "EOF?"=w372:bool)  [unwired: 4 in, 4 out]
      }
      n162 = call "Convert from Dynamic Data"("Dynamic Data Type"=w370) -> ("Array"=w362:dbl[][])  [unwired: 3 in]
      n163 = Array Subset(array=w362, index (row)=20 ("index"), length (row)=10 ("length")) -> (w367:dbl[][])  [unwired: 2 in]
      n164 = Array Subset(array=w362, index (row)=10 ("index"), length (row)=10 ("length")) -> ()  [unwired: 2 in, 1 out]
      n165 = Array Subset(array=w362, index (row)=0 ("index"), length (row)=10 ("length")) -> ()  [unwired: 2 in, 1 out]
      n166 = Array Subset(array=w362, index (row)=30 ("index"), length (row)=8 ("length")) -> (w351:dbl[][])  [unwired: 2 in]
      n167 = property on="PumpSeq 4" class="Arr (strict)"("Val(Sgnl)"=w367) -> ()  [unwired: 2 in, 2 out]
      n168 = Index Array(array=w351, index (row)=2, index (col)=0 ("disabled index (col)")) -> ()  [unwired: 1 out]
      n169 = Index Array(array=w351, index (row)=4, index (col)=0 ("disabled index (col)")) -> ()  [unwired: 1 out]
      n170 = Index Array(array=w351, index (row)=0, index (col)=1 ("disabled index (col)")) -> ()  [unwired: 1 out]
      n171 = Index Array(array=w351, index (row)=1, index (col)=1 ("disabled index (col)")) -> ()  [unwired: 1 out]
    }
    n172 = Boolean To (0,1)(Boolean=w107) -> (0, 1=w106:i16)
    n173 = for {
      N: w106 -> [_]
      n174 = property on="PAUSE/RUN 3" class="Bool (strict)"("Val(Sgnl)"=FALSE ("Value (Signaling)")) -> ()  [unwired: 2 in, 2 out]
    }
    n175 = Merge Signals(w265, w266, w216) -> (w223:dynamicdata)
    n176 = call "Build Table"("Include time data"=TRUE, "Signals"=w223) -> ("Table"=w277:string[][])  [unwired: 3 in, 6 out]
    n177 = Boolean To (0,1)(Boolean="PAUSE/RUN 5") -> (0, 1=w77:i16)
    n178 = for {
      N: w77 -> [_]
      tunnel: "MASTER CONTROL" -> [w292]
      tunnel: "PAUSE/RUN 5" -> [w291]
      n179 = And(x=w291, y="?") -> (x .and. y?=w300:bool)
      n180 = dll-call lib="C:/Users/shresplab/OneDrive - Kemira Oyj/Documents/GitHub/Bertta/BERTTA/x64/Debug/BERTTA.dll" fn="mettler"("port"="Scale port", "msg"=1) -> ("return type"=w294:dbl)  [unwired: 5 in, 2 out]
      n181 = And(x=w292, y=w300) -> (x .and. y?=w297:bool)
      n182 = Initialize Array(FALSE, 1 ("dimension size")) -> (w299:bool[])
      n183 = Replace Array Subset(array=w299, new element=w297, index=0) -> (w296:bool[])
      n184 = call "Convert to Dynamic Data5"("Double"=w294) -> ("Dynamic Data Type"=→"Waveform Chart 15":dynamicdata)  [unwired: 3 in]
      n185 = call "DAQ Assistant"("data"=w296, "device name"="CDAQ PAM Control") -> ()  [unwired: 16 in, 2 out]
    }
    n186 = Delete From Array(array=w277, length=13, index (col)=0 ("index (row)")) -> (array with subset deleted=→"Table":string[][])  [unwired: 1 in, 1 out]
    n187 = call "filenameparser_09.vi"("Description"="Description", "start path"="Browse folder", "Project name"="Project name", "User (initials)"="User (initials)", "OK Button in"="OK Button 2") -> ("appended path 2"=w239:path, "appended path"=w273:path)  [unwired: 4 in, 1 out]
    "Output File" <- w239
    n188 = Boolean To (0,1)(Boolean="OK Button") -> (0, 1=w272:i16)
    n189 = for {
      N: w272 -> [_]
      tunnel: w273 -> [w341]
      w345 = " " ("string")
      n190 = property on="Add comment" class="Str"("Val(Sgnl)"="" ("Value (Signaling)")) -> ()  [unwired: 2 in, 2 out]
      n191 = Get Date/Time String(want seconds? (F)=TRUE) -> (date string=w348:string, time string=w346:string)  [unwired: 2 in]
      n192 = Concatenate Strings(w348, w345, w346, w345, "Add comment") -> (w344:string)
      n193 = feedback #6() -> (w343:string[])  [unwired: 1 in]
      n194 = Build Array (concatenate)(w343, w344) -> (w342:string[])
      n195 = feedback-in #6(w342) -> ()
      n196 = Write to Text File(file (use dialog)=w341, text=w342) -> ()  [unwired: 2 in, 3 out]
    }
    n197 = call "Header Names 4.vi"("Dynamic Data"=w223) -> ("Signals Out"=w224:dynamicdata)  [unwired: 10 in]
    n198 = call "Write To Measurement File"("Signals"=w224, "Enable"="OK Button 2", "Filename"=w239) -> ()  [unwired: 14 in, 3 out]
    "Boolean" <- "OK Button 2"
  }
